vi "Graphics-Marker Text.vi"(0 "XYGraph":refnum<vi>, 5 "Slider":refnum<vi>, 9 "Text Labels[]":string[](array[string]), 11 "error in (no error)":errorcluster) -> (15 "error out":errorcluster)   [LabVIEW 2020]
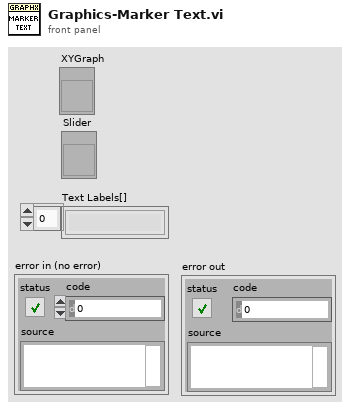
[diagram p1: front panel]
types:
  T1 = typedef "LVRangeTypeDef.ctl" = cluster{"Minimum":dbl, "Maximum":dbl, "Increment":dbl, "Minor Increment":dbl, "Start":dbl}
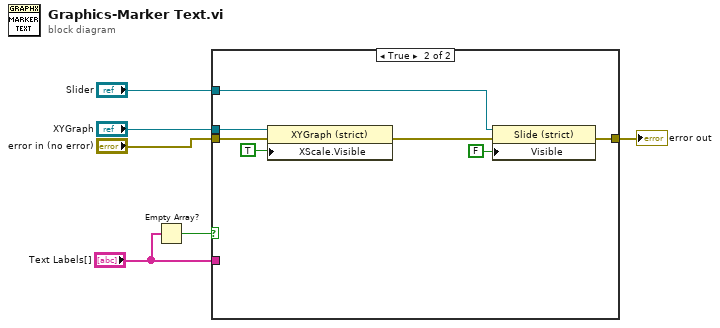
[diagram p0: block diagram]
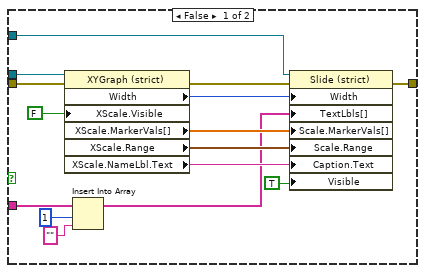
[diagram p2: hidden frame]
diagram:
  n1 = Empty Array?(array="Text Labels[]") -> (empty?=w1:bool)
  n2 = case shown="True" w1 {
    tunnel: "XYGraph" -> [w18 w28]
    tunnel: "Slider" -> [w17 w27]
    tunnel: [w15 w24] -> w4
    tunnel: "error in (no error)" -> [w14 w23]
    tunnel: "Text Labels[]" -> [w9 _]
    frame False {
      n3 = property on="Property Node" class="XYGraph (strict)"(reference=w18, error in=w14, "XScale.Visible"=FALSE ("Visible")) -> (error out=w16:errorcluster, "Width"=w21:u32, "XScale.MarkerVals[]"=w13:dbl[], "XScale.Range"=w20:T1, "XScale.NameLbl.Text"=w19:string)  [unwired: 1 out]
      n4 = Insert Into Array(array=w9, index=1, new element="" ("new element/subarray")) -> (w10:string[])
      n5 = property on="Property Node" class="Slide (strict)"(reference=w17, error in=w16, "Width"=w21, "TextLbls[]"=w10, "Scale.MarkerVals[]"=w13, "Scale.Range"=w20, "Caption.Text"=w19, "Visible"=TRUE) -> (error out=w15:errorcluster)  [unwired: 1 out]
    }
    frame True {
      n6 = property on="Property Node" class="XYGraph (strict)"(reference=w28, error in=w23, "XScale.Visible"=TRUE ("Visible")) -> (error out=w25:errorcluster)  [unwired: 1 out]
      n7 = property on="Property Node" class="Slide (strict)"(reference=w27, error in=w25, "Visible"=FALSE) -> (error out=w24:errorcluster)  [unwired: 1 out]
    }
  }
  "error out" <- w4
